vi "Filter_File_Type.vi"(8 "error in (no error)":errorcluster, 10 "file types":string[](array[string])=["exe", "bat"], 11 "IB_Source_Container in":refnum<class "IB_Source_Container.lvclass">) -> (0 "error out":errorcluster, 2 "pass?":bool, 3 "filtered model":refnum<class "IB_Source.lvclass">)   [LabVIEW 2020, in "IB_Source_Container.lvclass"]
uses:
  <vilib>/AppBuilder/IB_Classes/Source/Container/IB_Source_Container.lvclass
  <vilib>/AppBuilder/IB_Classes/Source/Container/IB_Source_Container.lvclass/IB_Source_Container.ctl
  <vilib>/AppBuilder/IB_Classes/Source/File/CtrFile/IB_CtrFile.lvclass
  e:/builds/penguin/labview/branches/2020/dev/dist/vi.lib/AppBuilder/IB_Classes/Source/IB_Source.lvclass
  e:/builds/penguin/labview/branches/2020/dev/dist/vi.lib/AppBuilder/IB_Classes/Source/Container/IB_Source_Container.lvclass
  <vilib>/AppBuilder/IB_Classes/Source/IB_Source.lvclass
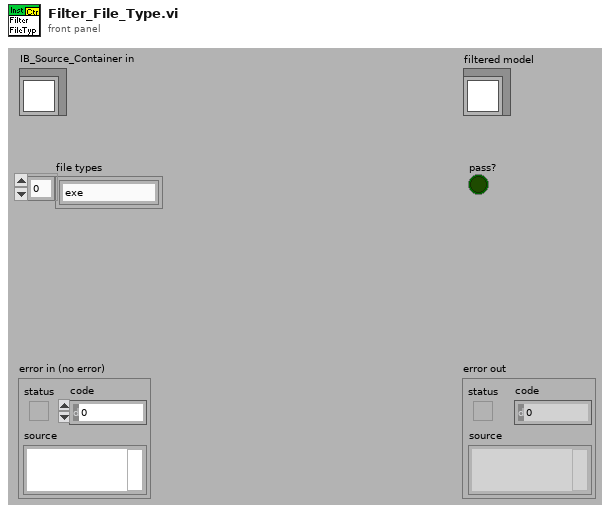
[diagram p1: front panel]
types:
  T1 = typedef "IB_Source_Container.ctl" = cluster{"files":refnum<class "IB_CtrFile.lvclass">[], "previewed?":bool, "preview error?":bool}
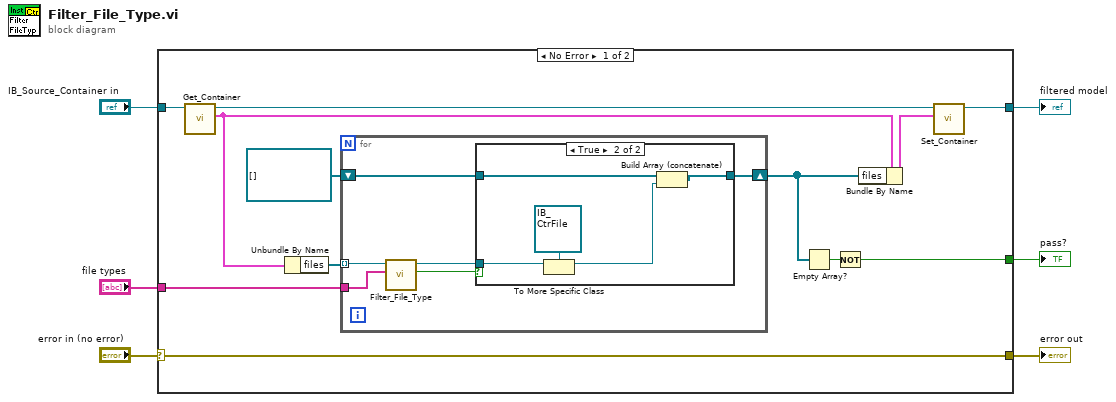
[diagram p0: block diagram]
diagram:
  n1 = case shown="No Error" "error in (no error)" {
    selector: "error in (no error)" -> [w14 w32]
    tunnel: "IB_Source_Container in" -> [w16 w31]
    tunnel: [w7 w31] -> w5
    tunnel: "file types" -> [w15 _]
    tunnel: [w14 w32] -> w2
    tunnel: [w12 _] -> w1
    frame No Error {
      n2 = call <vilib>:"Get_Container.vi"("IB_Source_Container in"=w16) -> ("data"=w11:T1, "IB_Source_Container out"=w8:refnum<class "IB_Source_Container.lvclass">)  [unwired: 1 in, 8 out]
      n3 = Unbundle By Name(w11) -> ("files"=w18:refnum<class "IB_CtrFile.lvclass">[])
      n4 = for {
        tunnel: w18 -> [w21] mode=indexing
        shift-right: [w23] -> w9
        shift-left: refnum<class "IB_CtrFile.lvclass">[] [] -> [w24]
        tunnel: w15 -> [w19]
        n5 = call-dynamic "Filter_File_Type.vi"("file types"=w19, "IB_Source_File in"=w21) -> ("pass?"=w22:bool, "filtered model"=w20:refnum<class "IB_Source.lvclass">)  [unwired: 1 in, 7 out]
        n6 = case shown="True" w22 {
          tunnel: w20 -> [_ w27]
          tunnel: w24 -> [w25 w30]
          tunnel: [w25 w29] -> w23
          frame False {
          }
          frame True {
            n7 = To More Specific Class(target class=refnum<class "IB_CtrFile.lvclass"> refnum ("IB_Source in"), reference=w27) -> (specific class reference=w26:refnum<class "IB_CtrFile.lvclass">)  [unwired: 1 in, 1 out]
            n8 = Build Array (concatenate)(w30, w26) -> (w29:refnum<class "IB_CtrFile.lvclass">[])
          }
        }
      }
      n9 = Empty Array?(array=w9) -> (empty?=w13:bool)
      n10 = Not(x=w13) -> (.not. x?=w12:bool)
      n11 = Bundle By Name(cluster=w11, "files"=w9) -> (w10:T1)
      n12 = call <vilib>:"Set_Container.vi"("data"=w10, "IB_Source_Container in"=w8) -> ("IB_Source_Container out"=w7:refnum<class "IB_Source_Container.lvclass">)  [unwired: 1 in, 8 out]
    }
    frame Error {
    }
  }
  "error out" <- w2
  "filtered model" <- w5
  "pass?" <- w1
